vi "NEWEST PI_0.vi"(0 "CtrlIndex":i32, 1 "ControlArray":T1(array[cluster]), 5 "CommandCluster":T3, 6 "Run?":bool, 7 "Feedback":dbl[](array[numeric]), 9 "VandPLimits":dbl[](array[numeric]), 11 "Stability In":T2, 12 "Tolerances":dbl[](array[numeric]), 13 "Controller?":bool, 14 "Ave Feedback":dbl[](array[numeric])) -> (4 "PIdata":dbl[](array[numeric]), 8 "Output":dbl, 10 "Stable?":bool, 15 "Stability Out":T2)   [LabVIEW 2013]
uses:
  TypeDef/Command Cluster.ctl
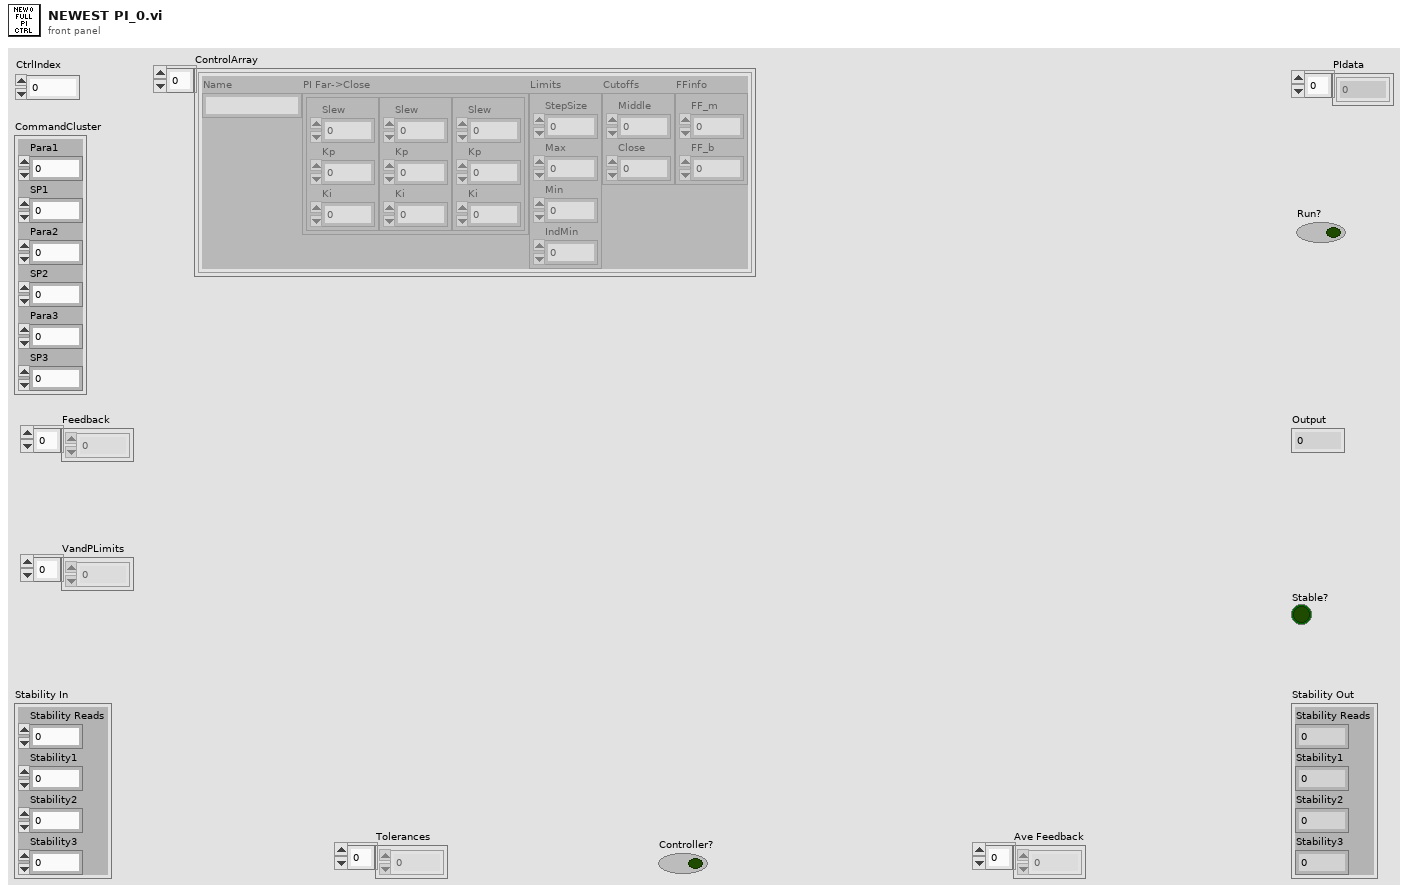
[diagram p1: front panel]
types:
  T1 = cluster{"Name":string, "PI Far->Close":cluster{"Slew":dbl, "Kp":dbl, "Ki":dbl}[], "Limits":cluster{"StepSize":dbl, "Max":dbl, "Min":dbl, "IndMin":dbl}, "Cutoffs":cluster{"Middle":dbl, "Close":dbl}, "FFinfo":cluster{"FF_m":dbl, "FF_b":dbl}}[]
  T2 = cluster{"Stability Reads":i32, "Stability1":i32, "Stability2":i32, "Stability3":i32}
  T3 = typedef "Command Cluster.ctl" = cluster{"Para1":i32, "SP1":dbl, "Para2":i32, "SP2":dbl, "Para3":i32, "SP3":dbl}
  T4 = cluster{"Name":string, "PI Far->Close":cluster{"Slew":dbl, "Kp":dbl, "Ki":dbl}[], "Limits":cluster{"StepSize":dbl, "Max":dbl, "Min":dbl, "IndMin":dbl}, "Cutoffs":cluster{"Middle":dbl, "Close":dbl}, "FFinfo":cluster{"FF_m":dbl, "FF_b":dbl}}
  T5 = cluster{"StepSize":dbl, "Max":dbl, "Min":dbl, "IndMin":dbl}
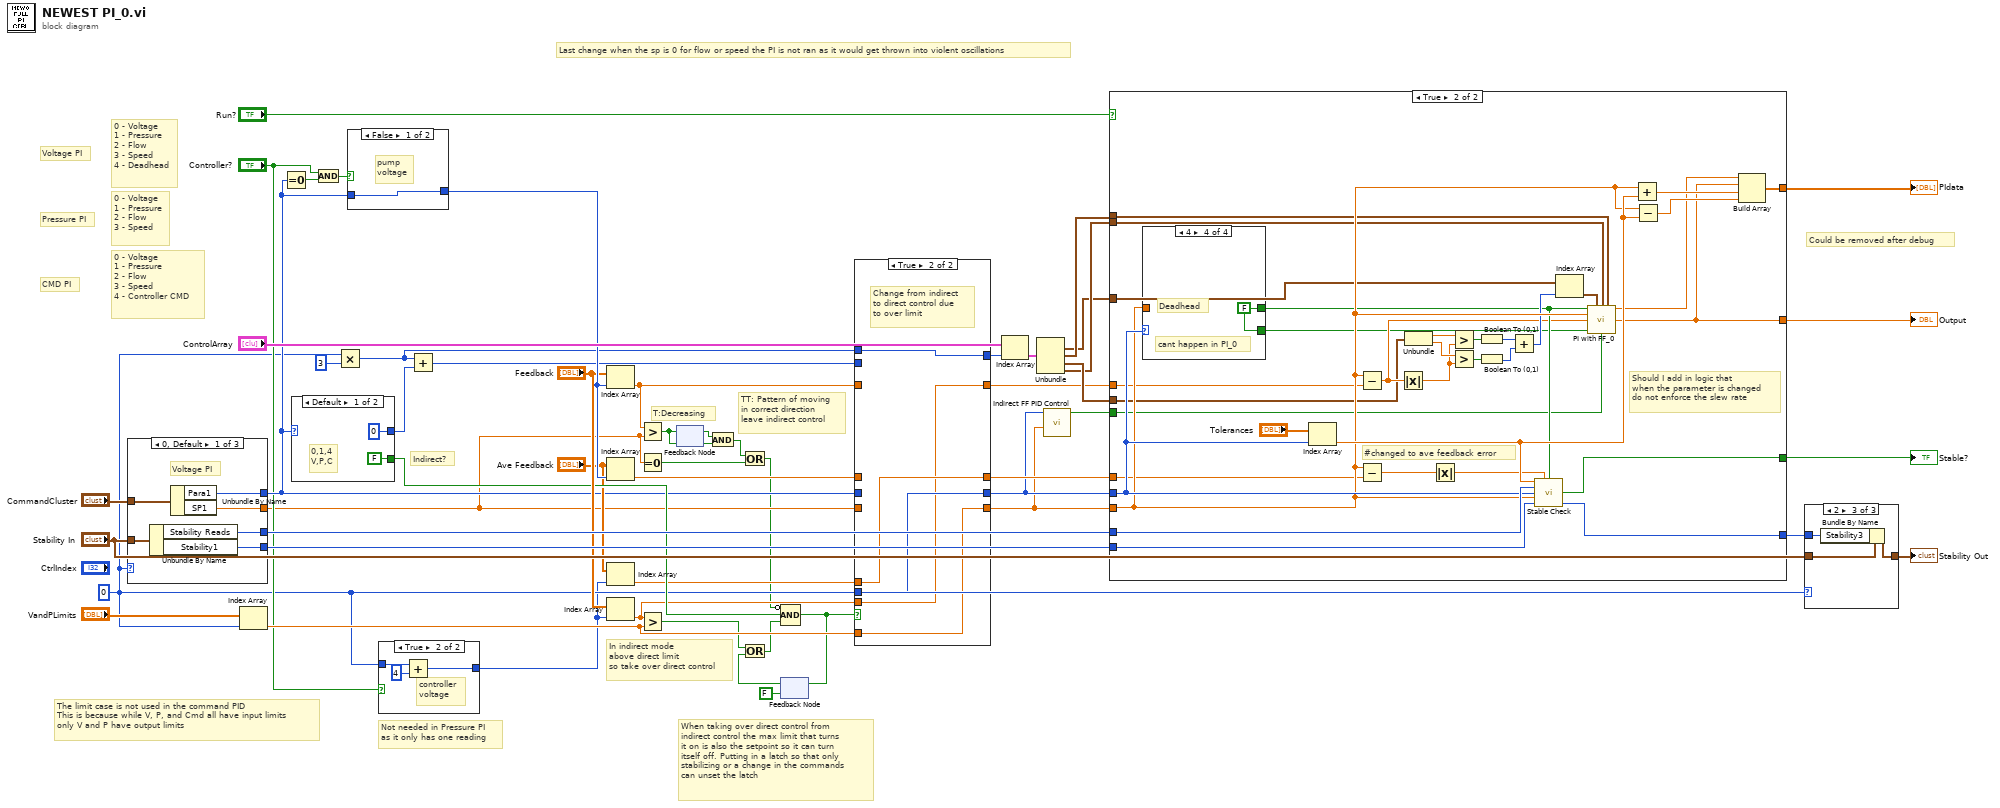
[diagram p0: block diagram]
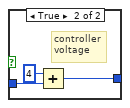
[diagram p4: hidden frame]
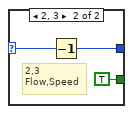
[diagram p5: hidden frame]
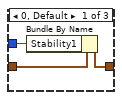
[diagram p6: hidden frame]
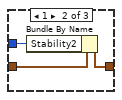
[diagram p7: hidden frame]
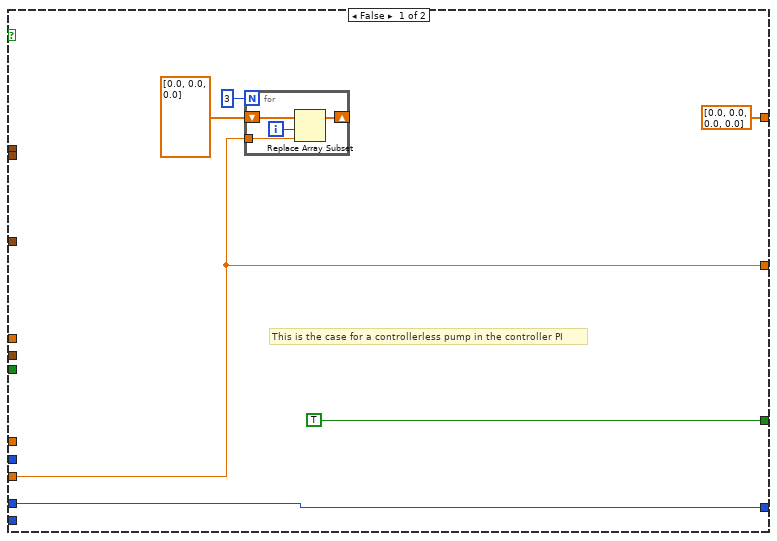
[diagram p8: hidden frame]
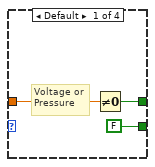
[diagram p9: hidden frame]
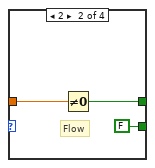
[diagram p10: hidden frame]
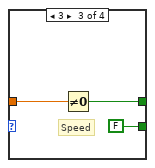
[diagram p11: hidden frame]
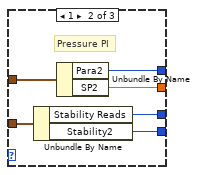
[diagram p12: hidden frame]
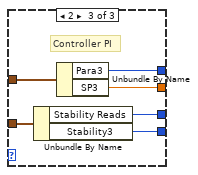
[diagram p13: hidden frame]
diagram:
  w14 = 0 ("CtrlIndex")
  # "When taking over direct control from\nindirect control the max limit that turns\nit on is also the setpoint so it can turn\nitself off. Putting in a latch so that only\nstabilizing or a change in the commands\ncan unset the latch"
  # "Not needed in Pressure PI\nas it only has one reading"
  # "TT: Pattern of moving\nin correct direction\nleave indirect control"
  # "In indirect mode\nabove direct limit\nso take over direct control"
  # "T:Decreasing"
  # "The limit case is not used in the command PID\nThis is because while V, P, and Cmd all have input limits\nonly V and P have output limits"
  # "Indirect?"
  # "Last change when the sp is 0 for flow or speed the PI is not ran as it would get thrown into violent oscillations"
  # "Could be removed after debug"
  # "CMD PI"
  # "Pressure PI"
  # "Voltage PI"
  # "0 - Voltage\n1 - Pressure\n2 - Flow\n3 - Speed\n4 - Controller CMD"
  # "0 - Voltage\n1 - Pressure\n2 - Flow\n3 - Speed"
  # "0 - Voltage\n1 - Pressure\n2 - Flow\n3 - Speed\n4 - Deadhead"
  n1 = case shown="0, Default" w14 {
    tunnel: "Stability In" -> [w59 w65 w71]
    tunnel: [w57 w63 w69] -> w52
    tunnel: [w58 w64 w70] -> w51
    tunnel: "CommandCluster" -> [w56 w62 w68]
    tunnel: [w54 w60 w67] -> w26
    tunnel: [w55 w61 w66] -> w12
    frame 0, Default {
      # "Voltage PI"
      n2 = Unbundle By Name(w59) -> ("Stability Reads"=w57:i32, "Stability1"=w58:i32)
      n3 = Unbundle By Name(w56) -> ("Para1"=w54:i32, "SP1"=w55:dbl)
    }
    frame 1 {
      # "Pressure PI"
      n4 = Unbundle By Name(w65) -> ("Stability Reads"=w63:i32, "Stability2"=w64:i32)
      n5 = Unbundle By Name(w62) -> ("Para2"=w60:i32, "SP2"=w61:dbl)
    }
    frame 2 {
      # "Controller PI"
      n6 = Unbundle By Name(w71) -> ("Stability Reads"=w69:i32, "Stability3"=w70:i32)
      n7 = Unbundle By Name(w68) -> ("Para3"=w67:i32, "SP3"=w66:dbl)
    }
  }
  n8 = Index Array(array="VandPLimits", index=w14) -> (element=w17:dbl)
  n9 = Equal To 0?(x=w26) -> (x = 0?=w34:bool)
  n10 = case shown="Default" w26 {
    selector: w26 -> [_ w76]
    tunnel: [0 w75] -> w36
    tunnel: [FALSE TRUE] -> w28
    frame Default {
      # "0,1,4\nV,P,C"
    }
    frame 2, 3 {
      # "2,3\nFlow,Speed"
      n11 = Decrement(x=w76) -> (x-1=w75:i32)
    }
  }
  n12 = And(x="Controller?", y=w34) -> (x .and. y?=w35:bool)
  n13 = Multiply(x=w14, y=3) -> (x*y=w16:i32)
  n14 = case shown="False" w35 {
    tunnel: w26 -> [w77 w80]
    tunnel: [w77 w78] -> w32
    frame False {
      # "pump\nvoltage"
    }
    frame True {
      # "controller\nvoltage"
      n15 = Add(x=4, y=w80) -> (x+y=w78:i32)
    }
  }
  n16 = case shown="True" "Controller?" {
    tunnel: [w81 w84] -> w13
    tunnel: w14 -> [w81 w83]
    frame False {
      # "pump\nvoltage"
    }
    frame True {
      # "controller\nvoltage"
      n17 = Add(x=w83, y=4) -> (x+y=w84:i32)
    }
  }
  n18 = Add(x=w16, y=w36) -> (x+y=w21:i32)
  n19 = Index Array(array="Feedback", index=w32) -> (element=w23:dbl)
  n20 = Index Array(array="Ave Feedback", index=w32) -> (element=w25:dbl)
  n21 = Index Array(array="Ave Feedback", index=w13) -> (element=w19:dbl)
  n22 = Index Array(array="Feedback", index=w13) -> (element=w18:dbl)
  n23 = Greater?(x=w23, y=w12) -> (0:w29:bool)
  n24 = Equal To 0?(x=w12) -> (x = 0?=w11:bool)
  n25 = Greater?(x=w18, y=w17) -> (0:w5:bool)
  n26 = feedback-in #1(w29) -> ()
  n27 = feedback #1(w29) -> (w30:bool)
  n28 = And(x=w30, y=w29) -> (x .and. y?=w10:bool)
  n29 = Or(x=w10, y=w11) -> (x .or. y?=w9:bool)
  n30 = feedback #2(FALSE) -> (w6:bool)
  n31 = Or(x=w5, y=w6) -> (x .or. y?=w4:bool)
  n32 = Compound Arithmetic op=AND(invert w9, w28, w4) -> (w8:bool)
  n33 = feedback-in #2(w8) -> ()
  n34 = case shown="True" w8 {
    tunnel: w26 -> [w88 _]
    tunnel: w12 -> [w87 _]
    tunnel: [w88 w93] -> w3
    tunnel: [w87 w94] -> w2
    tunnel: w25 -> [w89 _]
    tunnel: [w89 w92] -> w24
    tunnel: w23 -> [w86 _]
    tunnel: [w86 w91] -> w22
    tunnel: w21 -> [w85 _]
    tunnel: [w85 w90] -> w20
    tunnel: w19 -> [_ w92]
    tunnel: w18 -> [_ w91]
    tunnel: w17 -> [_ w94]
    tunnel: w14 -> [_ w93]
    tunnel: w16 -> [_ w90]
    frame False {
      # "Leave controls as is"
    }
    frame True {
      # "Change from indirect\nto direct control due\nto over limit"
    }
  }
  n35 = Index Array(array="ControlArray", index=w20) -> (element=w41:T4)
  n36 = Unbundle(w41) -> ("PI Far->Close"=w37:cluster{"Slew":dbl, "Kp":dbl, "Ki":dbl}[], "Limits"=w38:T5, "Cutoffs"=w40:cluster{"Middle":dbl, "Close":dbl}, "FFinfo"=w39:cluster{"FF_m":dbl, "FF_b":dbl})  [unwired: 1 out]
  n37 = call "Indirect FF PID Control.vi"("Setpoint"=w2, "Parameter"=w3) -> ("Indirect FF"=w1:bool)  [unwired: 9 in]
  n38 = case shown="True" "Run?" {
    tunnel: w52 -> [w99 w129]
    tunnel: w51 -> [_ w128]
    tunnel: w3 -> [_ w127]
    tunnel: w2 -> [w98 w121]
    tunnel: [TRUE w124] -> w49
    tunnel: [w98 w109] -> w48
    tunnel: [dbl[] [0.0, 0.0, 0.0, 0.0] w137] -> w47
    tunnel: [w99 w130] -> w46
    tunnel: w38 -> [_ w113]
    tunnel: w40 -> [_ w112]
    tunnel: w39 -> [_ w111]
    tunnel: w37 -> [_ w110]
    tunnel: w22 -> [_ w107]
    tunnel: w24 -> [_ w106]
    tunnel: w1 -> [_ w105]
    frame False {
      # "This is the case for a controllerless pump in the controller PI"
      n39 = for {
        N: 3 -> [_]
        shift-right: [w103] -> _
        shift-left: dbl[] [0.0, 0.0, 0.0] -> [w104]
        tunnel: w98 -> [w101]
        i -> [w102]
        n40 = Replace Array Subset(array=w104, new element=w101, index=w102) -> (w103:dbl[])
      }
    }
    frame True {
      # "#changed to ave feedback error"
      # "Should I add in logic that\nwhen the parameter is changed\ndo not enforce the slew rate"
      n41 = case shown="4" w127 {
        tunnel: [w139 w143 w146 w148] -> w117
        tunnel: w121 -> [w140 w144 w147 _]
        tunnel: [FALSE FALSE FALSE w148] -> w115
        frame Default {
          # "Voltage or\nPressure"
          n42 = Not Equal To 0?(x=w140) -> (x != 0?=w139:bool)
        }
        frame 2 {
          # "Flow"
          n43 = Not Equal To 0?(x=w144) -> (x != 0?=w143:bool)
        }
        frame 3 {
          # "Speed"
          n44 = Not Equal To 0?(x=w147) -> (x != 0?=w146:bool)
        }
        frame 4 {
          w148 = FALSE
          # "cant happen in PI_0"
          # "Deadhead"
        }
      }
      n45 = Index Array(array="Tolerances", index=w127) -> (element=w123:dbl)
      n46 = Subtract(x=w121, y=w107) -> (x-y=w116:dbl)
      n47 = Subtract(x=w121, y=w106) -> (x-y=w126:dbl)
      n48 = Absolute Value(x=w116) -> (abs(x)=w125:dbl)
      n49 = Unbundle(w112) -> ("Middle"=w132:dbl, "Close"=w131:dbl)
      n50 = Absolute Value(x=w126) -> (abs(x)=w122:dbl)
      n51 = Greater?(x=w132, y=w125) -> (0:w136:bool)
      n52 = Greater?(x=w131, y=w125) -> (0:w135:bool)
      n53 = Boolean To (0,1)(Boolean=w136) -> (0, 1=w134:i16)
      n54 = Boolean To (0,1)(Boolean=w135) -> (0, 1=w133:i16)
      n55 = Add(x=w134, y=w133) -> (x+y=w118:i16)
      n56 = call "Stable Check.vi"("Tolerance"=w123, "AbsError"=w122, "PI Running?"=w117, "ReqReads"=w129, "Parameter"=w127, "Setpoint"=w121, "StabilityCount In"=w128) -> ("Stable?"=w124:bool, "StabilityCount Out"=w130:i32)  [unwired: 6 in, 1 out]
      n57 = Index Array(array=w110, index=w118) -> (element=w114:cluster{"Slew":dbl, "Kp":dbl, "Ki":dbl})
      n58 = call "PI with FF_0.vi"("Run PI?"=w117, "PIcluster"=w114, "FFcluster"=w111, "LimitCluster"=w113, "SP"=w121, "Error"=w116, "RevCtrlZero"=w115, "Indirect FF"=w105) -> ("PreSlew"=w108:dbl, "Output"=w109:dbl)  [unwired: 6 in]
      n59 = Add(x=w121, y=w123) -> (x+y=w120:dbl)
      n60 = Subtract(x=w121, y=w123) -> (x-y=w119:dbl)
      n61 = Build Array(w108, w109, w120, w119) -> (w137:dbl[])
    }
  }
  "Stable?" <- w49
  "Output" <- w48
  "PIdata" <- w47
  n62 = case shown="2" w14 {
    tunnel: "Stability In" -> [w150 w153 w156]
    tunnel: [w149 w152 w155] -> w50
    tunnel: w46 -> [w151 w154 w157]
    frame 0, Default {
      n63 = Bundle By Name(cluster=w150, "Stability1"=w151) -> (w149:T2)
    }
    frame 1 {
      n64 = Bundle By Name(cluster=w153, "Stability2"=w154) -> (w152:T2)
    }
    frame 2 {
      n65 = Bundle By Name(cluster=w156, "Stability3"=w157) -> (w155:T2)
    }
  }
  "Stability Out" <- w50
